vi "espectro_discreto_db.vi"(11 "Filtered X":dbl[](array[numeric])) -> (1 "DFT dB":dbl[](array[numeric]), 2 "DFT":dbl[](array[numeric]), 3 "Multiplier factor":dbl)   [LabVIEW 2020]
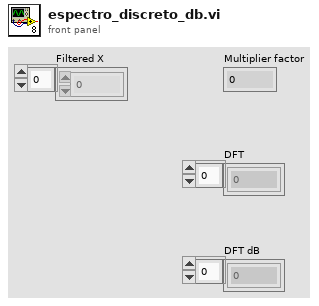
[diagram p1: front panel]
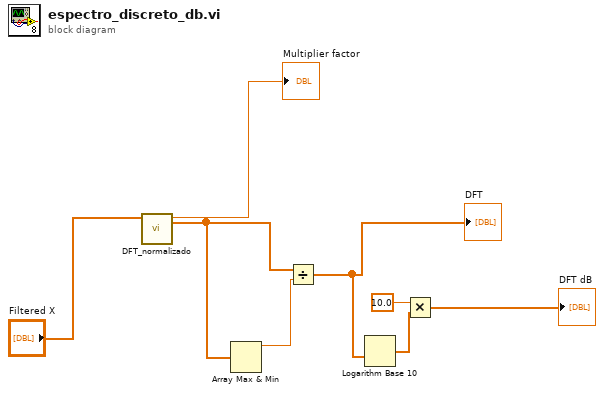
[diagram p0: block diagram]
diagram:
  n1 = call "DFT_normalizado.vi"("X"="Filtered X") -> ("Array"=w3:dbl[], "Numeric"=→"Multiplier factor":dbl)  [unwired: 9 in]
  n2 = Array Max & Min(array=w3) -> (max value=w2:dbl)  [unwired: 3 out]
  n3 = Divide(x=w3, y=w2) -> (x/y=w6:dbl[])
  "DFT" <- w6
  n4 = Logarithm Base 10(1:w6) -> (0:w5:dbl[])
  n5 = Multiply(x=10.0, y=w5) -> (x*y=→"DFT dB":dbl[])
